vi "peak_detection.vi"() -> ()   [LabVIEW 2019]
uses:
  <vilib>/Utility/file.llb/Read Delimited Spreadsheet (DBL).vi
  <vilib>/Utility/file.llb/Write Delimited Spreadsheet (DBL).vi
panel:
  in  "執行":bool
  out "Mark point":cluster{"X":dbl, "Y":dbl}[](array[cluster])
  in  "Point mark file":path
  in  "Signal file":path
  out "XY":cluster{"X":dbl, "Y":dbl}
  in  "Save":bool
  out "XY Graph":cluster{"all rows":dbl[], "all rows":dbl[]}[](graph)
  # "先選data檔，會自動設定anno檔路徑，若要另外指定路徑再自行設定"
  # "操作步驟\n\n1.選擇訊號檔案。\n2.可以讀取之前抓到一半的檔案，如果沒有選取系統會自動創一個。\n3.開始抓點，在R波頂端按下滑鼠左鍵即可抓點，欲刪除點雙擊左鍵。\n4.抓完檔案按下Save即完成抓點。"
  # "讀取之前未取完點的存檔       預設存檔會與signal file同一資料夾下      檔名: filename_anno"
  # "單擊新增點\n雙擊刪除最近的點"
  # "抓到的點的資料"
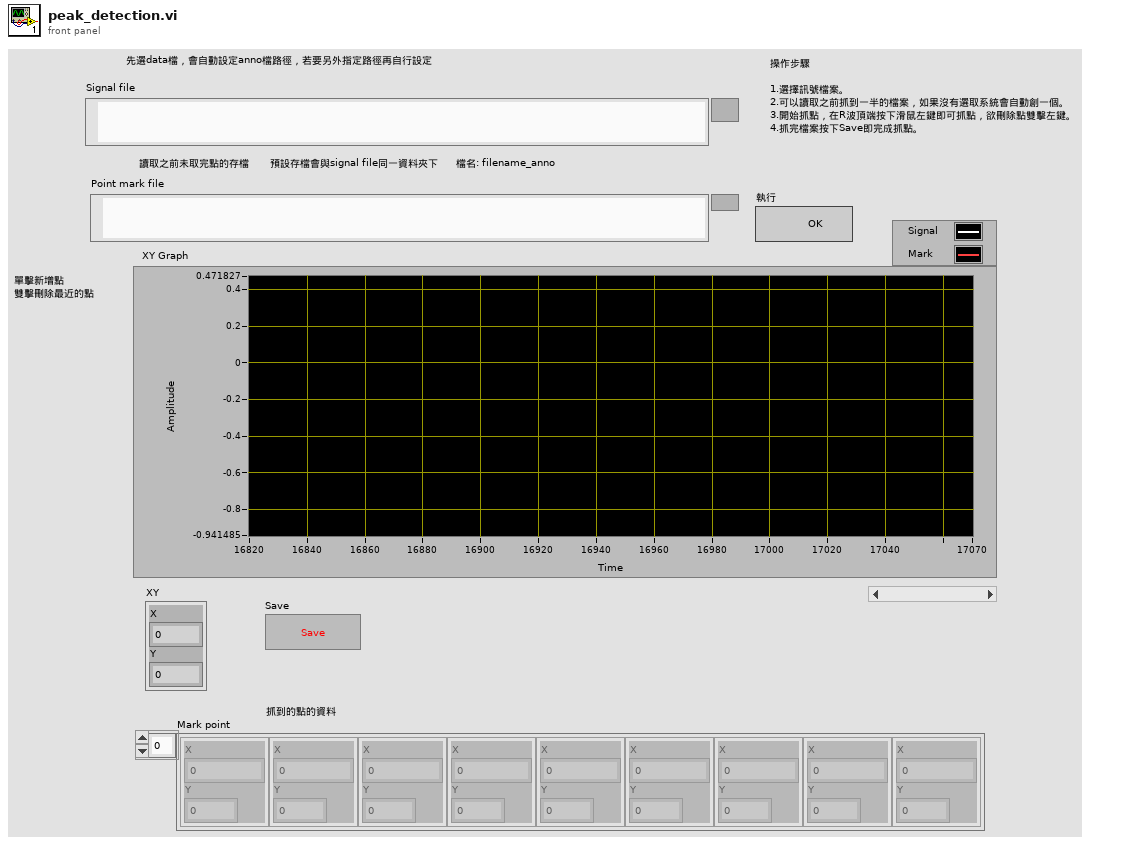
[diagram p1: front panel]
types:
  T1 = typedef "LVPoint32TypeDef.ctl" = cluster{"Horizontal":i32, "Vertical":i32}
  T2 = enum16{"open", "replace", "create", "open or create", "replace or create", "replace or create with confirmation"}
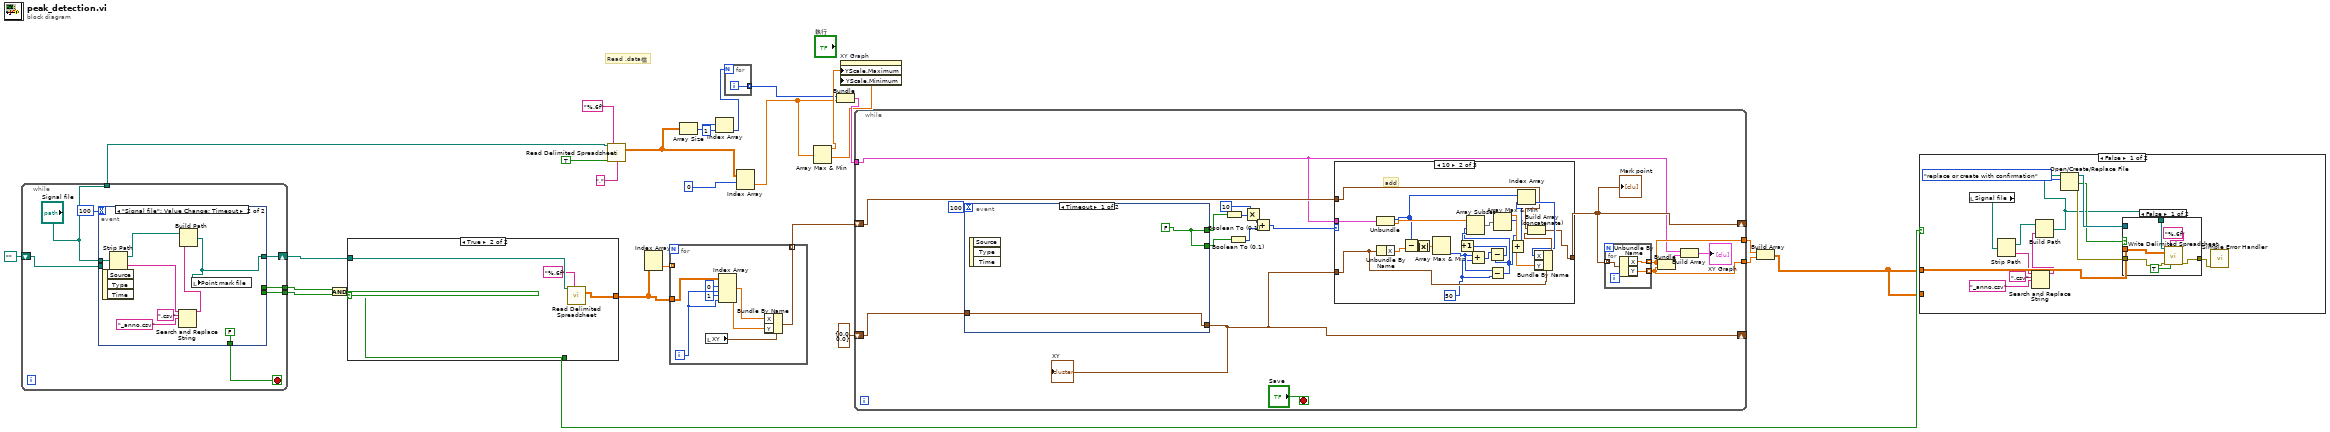
[diagram p0: block diagram]
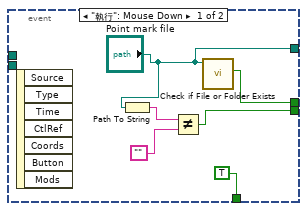
[diagram p2: hidden frame]
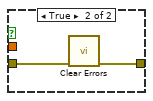
[diagram p3: hidden frame]
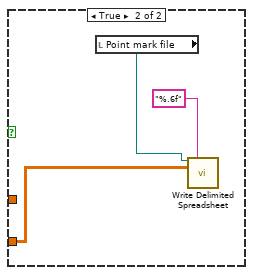
[diagram p4: hidden frame]
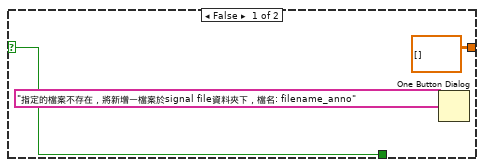
[diagram p5: hidden frame]
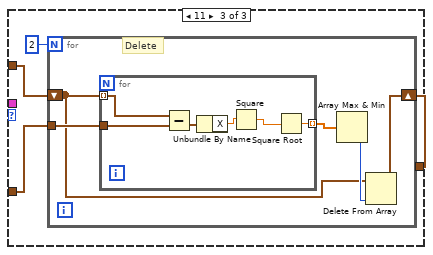
[diagram p7: hidden frame]
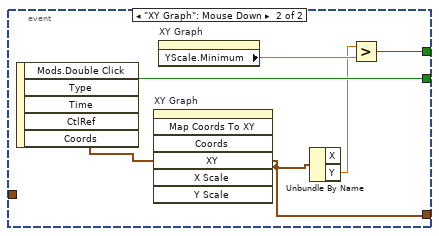
[diagram p8: hidden frame]
diagram:
  # "Read .data檔"
  n1 = while {
    tunnel: [w34] -> w19
    tunnel: [w33] -> w18
    tunnel: ["Signal file"] -> w9
    shift-right: [w30] -> w8
    shift-left: path "" ("appended path") -> [w28]
    stop <- w32 stop-if-true
    n2 = event shown="[1] \"Signal file\": Value Change;  Timeout" {
      selector: _ -> [_ _]
      dyn-events: _ -> [_ _]
      timeout: 100 -> [_ _]
      tunnel: [w38 _] -> w34
      tunnel: [w37 _] -> w33
      tunnel: ["Point mark file" w46] -> w30
      tunnel: [TRUE FALSE] -> w32
      tunnel: "Signal file" -> [_ w45]
      tunnel: w28 -> [_ _]
      event "執行": Mouse Down {
        n3 = event-data() -> ()  [unwired: 1 in, 7 out]
        n4 = Path To String(path="Point mark file") -> (string=w40:string)
        n5 = Not Equal?(x=w40, y="") -> (x != y?=w37:bool)
        n6 = call <vilib>:"Check if File or Folder Exists.vi"("path"="Point mark file") -> ("file or folder exists?"=w38:bool)  [unwired: 8 in, 2 out]
      }
      event "Signal file": Value Change; Timeout {
        n7 = event-data() -> ()  [unwired: 1 in, 3 out]
        n8 = Strip Path(path=w45) -> (stripped path=w48:path, name=w43:string)
        n9 = Search and Replace String(input string=w43, search string=".csv", replace string="_anno.csv" ("string")) -> (result string=w42:string)  [unwired: 5 in, 3 out]
        n10 = Build Path(base path=w48, name or relative path=w42) -> (appended path=w46:path)
        n11 = local write "Point mark file"(w46) -> ()
      }
    }
  }
  n12 = And(x=w19, y=w18) -> (x .and. y?=w17:bool)
  n13 = case shown="True" w17 {
    selector: w17 -> [w49 w52]
    tunnel: w8 -> [_ w55]
    tunnel: [dbl[][] [] ("all rows") w53] -> w13
    tunnel: [w49 w52] -> w11
    frame False {
      n14 = One Button Dialog(message="指定的檔案不存在，將新增一檔案於signal file資料夾下，檔名: filename_anno") -> ()  [unwired: 1 in, 1 out]
    }
    frame True {
      n15 = call-poly <vilib>:"Read Delimited Spreadsheet.vi"("file path (dialog if empty)"=w55, "format (%.3f)"="%.6f") -> ("all rows"=w53:dbl[][])  [unwired: 8 in, 5 out]
    }
  }
  n16 = call-poly <vilib>:"Read Delimited Spreadsheet.vi"("file path (dialog if empty)"=w9, "format (%.3f)"="%.6f" ("format (%d)"), "transpose? (F)"=TRUE, "delimiter (\\t)"="," ("delimiter (\\t)")) -> ("all rows"=w6:dbl[][])  [unwired: 6 in, 5 out]
  n17 = Index Array(array=w13) -> (element=w12:dbl[])  [unwired: 2 in]
  n18 = for {
    tunnel: w13 -> [w61]
    tunnel: [w62] -> w16 mode=indexing
    tunnel: w12 -> [_] mode=indexing
    i -> [w60]
    n19 = local read "XY"() -> (w63:cluster{"X":dbl, "Y":dbl})
    n20 = Index Array(array=w61, index (row) #1=0 ("disabled index (row)"), index (col) #1=w60, index (row) #2=1 ("disabled index (row)"), index (col) #2=w60) -> (element #1=w57:dbl, element #2=w56:dbl)
    n21 = Bundle By Name(cluster=w63, "X"=w57, "Y"=w56) -> (w62:cluster{"X":dbl, "Y":dbl})
  }
  n22 = Array Size(array=w6) -> (size(s)=w5:i32[])
  n23 = Index Array(array=w5, index=1) -> (element=w3:i32)
  n24 = for {
    N: w3 -> [_]
    tunnel: [w64] -> w2 mode=indexing
    i -> [w64]
  }
  n25 = Index Array(array=w6, index (row)=0) -> (element=w4:dbl[])  [unwired: 1 in]
  n26 = Array Max & Min(array=w4) -> (max value=w21:dbl, min value=w20:dbl)  [unwired: 2 out]
  n27 = Bundle(w2, "all rows"=w4) -> (w22:cluster{i32[], "all rows":dbl[]})  [unwired: 1 in]
  n28 = property on="XY Graph" class="XYGraph (strict)"("YScale.Maximum"=w21, "YScale.Minimum"=w20) -> ()  [unwired: 2 in, 2 out]
  n29 = while {
    shift-right: [w74] -> _
    shift-left: cluster{"X":dbl, "Y":dbl} {"X"=0.0, "Y"=0.0} ("XY") -> [w80]
    shift-right: [w66] -> _
    shift-left: w16 -> [w73]
    tunnel: w22 -> [w65]
    tunnel: [w68] -> w15
    tunnel: [w67] -> w14
    stop <- "Save" stop-if-true
    n30 = event shown="[0] Timeout" {
      selector: _ -> [_ _]
      dyn-events: _ -> [_ _]
      timeout: 100 -> [_ _]
      tunnel: [w124 w127] -> w74
      tunnel: w80 -> [w124 _]
      tunnel: [w123 w129] -> w78
      tunnel: [w123 w125] -> w79
      event Timeout {
        w123 = FALSE
        n31 = event-data() -> ()  [unwired: 1 in, 3 out]
      }
      event "XY Graph": Mouse Down {
        n32 = event-data() -> ("Mods.Double Click"=w129:bool, "Coords"=w130:T1)  [unwired: 1 in, 3 out]
        n33 = invoke on="XY Graph" class="XYGraph (strict)" method="Map Coords To XY"("Coords"=w130) -> ("XY"=w127:cluster{"X":dbl, "Y":dbl})  [unwired: 6 in, 6 out]
        n34 = property on="XY Graph" class="XYGraph (strict)"() -> ("YScale.Minimum"=w128:dbl)  [unwired: 2 in, 2 out]
        n35 = Unbundle By Name(w127) -> ("Y"=w126:dbl)  [unwired: 1 out]
        n36 = Greater?(x=w126, y=w128) -> (0:w125:bool)
      }
    }
    "XY" <- w74
    n37 = Boolean To (0,1)(Boolean=w79) -> (0, 1=w77:i16)
    n38 = Boolean To (0,1)(Boolean=w78) -> (0, 1=w76:i16)
    n39 = Multiply(x=w77, y=i16 10) -> (x*y=w72:i16)
    n40 = Add(x=w72, y=w76) -> (x+y=w75:i16)
    n41 = case shown="10" w75 {
      tunnel: w74 -> [_ w88 w111]
      tunnel: [w86 w91 w109] -> w66
      tunnel: w73 -> [w86 w90 w110]
      tunnel: w65 -> [_ w89 _]
      frame 0, Default {
      }
      frame 10 {
        w87 = 50 ("y")
        # "add"
        n42 = Unbundle(w89) -> (w96:i32[], "all rows"=w107:dbl[])
        n43 = Unbundle By Name(w88) -> ("X"=w106:dbl)
        n44 = Subtract(x=w96, y=w106) -> (x-y=w93:dbl[])
        n45 = Absolute Value(x=w93) -> (abs(x)=w92:dbl[])
        n46 = Array Max & Min(array=w92) -> (min index (indices)=w105:i32)  [unwired: 3 out]
        n47 = Add(x=w105, y=w87) -> (x+y=w104:i32)
        n48 = Subtract(x=w105, y=w87) -> (x-y=w99:i32)
        n49 = Subtract(x=w104, y=w99) -> (x-y=w103:i32)
        n50 = Increment(x=w103) -> (x+1=w102:i32)
        n51 = Array Subset(array=w107, index=w99, length=w102) -> (w101:dbl[])
        n52 = Array Max & Min(array=w101) -> (max value=w100:dbl, max index (indices)=w97:i32)  [unwired: 2 out]
        n53 = Add(x=w97, y=w99) -> (x+y=w95:i32)
        n54 = Index Array(array=w96, index=w95) -> (element=w94:i32)
        n55 = Bundle By Name(cluster=w88, "X"=w94, "Y"=w100) -> (w98:cluster{"X":dbl, "Y":dbl})
        n56 = Build Array (concatenate)(w90, w98) -> (w91:cluster{"X":dbl, "Y":dbl}[])
      }
      frame 11 {
        n57 = for {
          N: 2 -> [_]
          tunnel: w111 -> [w116]
          shift-right: [w112] -> w109
          shift-left: w110 -> [w113]
          # "Delete"
          n58 = for {
            tunnel: w113 -> [w122] mode=indexing
            tunnel: w116 -> [w121]
            tunnel: [w118] -> w115 mode=indexing
            n59 = Subtract(x=w122, y=w121) -> (x-y=w120:cluster{"X":dbl, "Y":dbl})
            n60 = Unbundle By Name(w120) -> ("X"=w119:dbl)
            n61 = Square(x=w119) -> (x^2=w117:dbl)
            n62 = Square Root(x=w117) -> (sqrt(x)=w118:dbl)
          }
          n63 = Array Max & Min(array=w115) -> (min index (indices)=w114:i32)  [unwired: 3 out]
          n64 = Delete From Array(array=w113, index=w114) -> (array with subset deleted=w112:cluster{"X":dbl, "Y":dbl}[])  [unwired: 1 in, 1 out]
        }
      }
    }
    "Mark point" <- w66
    n65 = for {
      tunnel: w66 -> [w85] mode=indexing
      tunnel: [w84] -> w68 mode=indexing
      tunnel: [w83] -> w67 mode=indexing
      n66 = Unbundle By Name(w85) -> ("X"=w84:dbl, "Y"=w83:dbl)
    }
    n67 = Bundle(w68, w67) -> (w70:cluster{dbl[], dbl[]})  [unwired: 1 in]
    n68 = Build Array(w65, w70) -> (→"XY Graph":cluster{dbl[], "all rows":dbl[]}[])
  }
  n69 = Build Array(w15, w14) -> (w10:dbl[][])
  n70 = case shown="False" w11 {
    tunnel: w10 -> [_ w152]
    tunnel: w10 -> [w136 _]
    frame False {
      n71 = local read "Signal file"() -> (w143:path)
      n72 = Strip Path(path=w143) -> (stripped path=w142:path, name=w134:string)
      n73 = Search and Replace String(input string=w134, search string=".csv", replace string="_anno.csv" ("string")) -> (result string=w131:string)  [unwired: 5 in, 3 out]
      n74 = Build Path(base path=w142, name or relative path=w131) -> (appended path=w135:path)
      n75 = Open/Create/Replace File(file path (use dialog)=w135, operation (0:open)=T2."replace or create with confirmation") -> (refnum out=w140:refnum<file>, cancelled=w139:bool, error out=w138:errorcluster)  [unwired: 4 in]
      n76 = case shown="False" w139 {
        tunnel: w140 -> [_ _]
        tunnel: w138 -> [w146 w151]
        tunnel: [w145 w150] -> w137
        tunnel: w136 -> [w148 _]
        tunnel: w135 -> [w147 _]
        frame False {
          n77 = call-poly <vilib>:"Write Delimited Spreadsheet.vi"("file path (dialog if empty)"=w147, "format (%.3f)"="%.6f", "2D data"=w148, "error in (no error)"=w146, "transpose? (no:F)"=TRUE) -> ("error out"=w145:errorcluster)  [unwired: 9 in, 1 out]
        }
        frame True {
          n78 = call <vilib>:"Clear Errors.vi"("error in (no error)"=w151) -> ("error out"=w150:errorcluster)  [unwired: 5 in, 1 out]
        }
      }
      n79 = call <vilib>:"Simple Error Handler.vi"("error in (no error)"=w137) -> ()  [unwired: 4 in, 5 out]
    }
    frame True {
      n80 = local read "Point mark file"() -> (w153:path)
      n81 = call-poly <vilib>:"Write Delimited Spreadsheet.vi"("file path (dialog if empty)"=w153, "format (%.3f)"="%.6f", "2D data"=w152) -> ()  [unwired: 11 in, 2 out]
    }
  }
